vi "Colour to HSL.vi"(8 "error in (no error)":errorcluster, 11 "Color":u32(colorbox)) -> (0 "error out":errorcluster, 1 "Lightness(%)":dbl format="%#_13g", 2 "Saturation(%)":dbl format="%#_13g", 3 "Hue(°)":dbl format="%#_13g", 5 "Resolved Color":u32 format="%.0x")   [LabVIEW 2018, in "Colour Lab.lvlib"]
uses:
  Colour Lab.lvlib
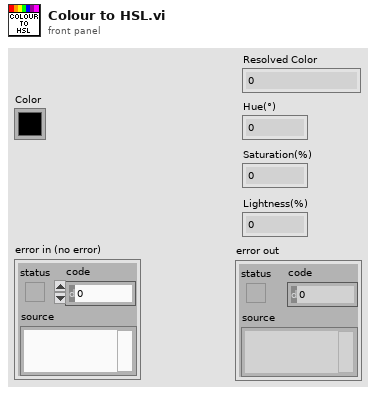
[diagram p1: front panel]
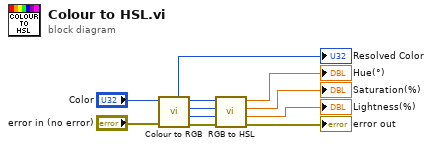
[diagram p0: block diagram]
diagram:
  n1 = call "Colour to RGB.vi"("error in (no error)"="error in (no error)", "Color"="Color") -> ("error out"=w11:errorcluster, "Blue"=w10:u8, "Green"=w9:u8, "Red"=w8:u8, "Resolved Color"=→"Resolved Color":u32)  [unwired: 5 in]
  n2 = call "RGB to HSL.vi"("error in (no error)"=w11, "Blue"=w10, "Green"=w9, "Red"=w8) -> ("error out"=→"error out":errorcluster, "Lightness(%)"=→"Lightness(%)":dbl, "Saturation(%)"=→"Saturation(%)":dbl, "Hue(°)"=→"Hue(°)":dbl)  [unwired: 4 in]
